vi "Idle Connection - Client.vi"(0 "connection ID":refnum<k5>, 3 "error in (no error)":errorcluster) -> (7 "connection ID out":refnum<k5>, 8 "Connection Established?":bool, 9 "Message from Server":string, 10 "No error":errorcluster)   [LabVIEW 2020]
doc: "Tests ports in direction of cliend to server"
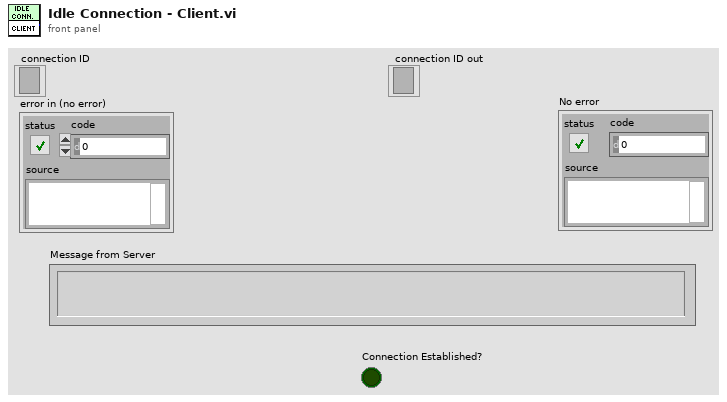
[diagram p1: front panel]
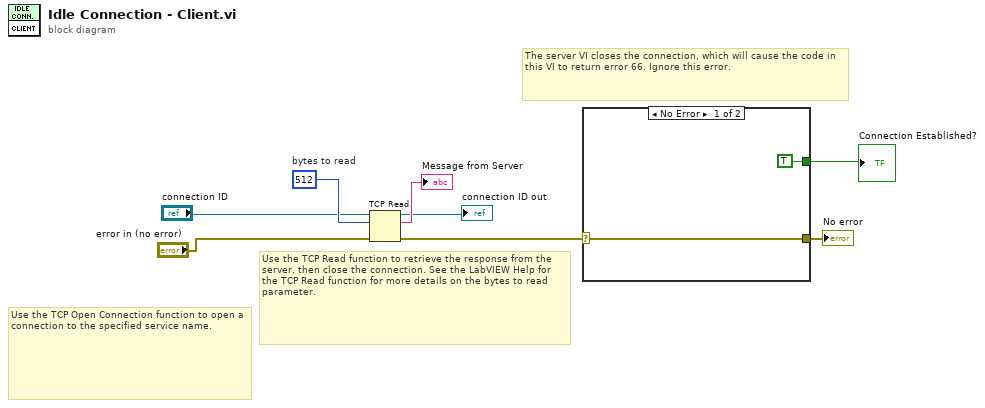
[diagram p0: block diagram]
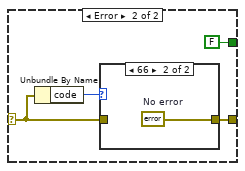
[diagram p2: hidden frame]
diagram:
  w6 = 512  # bytes to read
  # "The server VI closes the connection, which will cause the code in this VI to return error 66. Ignore this error."
  # "Use the TCP Open Connection function to open a connection to the specified service name."
  # "Use the TCP Read function to retrieve the response from the server, then close the connection. See the LabVIEW Help for the TCP Read function for more details on the bytes to read parameter."
  n1 = TCP Read(connection ID="connection ID", bytes to read=w6, error in (no error)="error in (no error)") -> (connection ID out=→"connection ID out":refnum<k5>, data out=→"Message from Server":string, error out=w8:errorcluster)  [unwired: 2 in]
  n2 = case shown="No Error" w8 {
    selector: w8 -> [w10 w13]
    tunnel: [w10 w12] -> w5
    tunnel: [TRUE FALSE] -> w4
    frame No Error {
    }
    frame Error {
      n3 = Unbundle By Name(w13) -> ("code"=w14:i32)
      n4 = case shown="66" w14 {
        tunnel: w13 -> [w15 _]
        tunnel: [w15 w16] -> w12
        frame Default {
        }
        frame 66 {
          w16 = errorcluster {"status"=FALSE, "code"=0, "source"=""}  # No error
        }
      }
    }
  }
  "No error" <- w5
  "Connection Established?" <- w4
